vi "Common-AddMsgToListBox.vi"(10 "字符串":string, 11 "列表框":refnum<vi>) -> ()   [LabVIEW 2014]
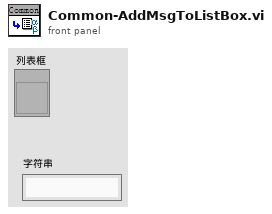
[diagram p1: front panel]
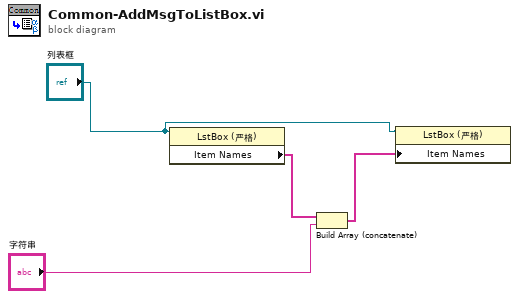
[diagram p0: block diagram]
diagram:
  n1 = property class="LstBox (严格)"(reference="列表框") -> ("Item Names"=w4:string[])  [unwired: 1 in, 2 out]
  n2 = Build Array (concatenate)(w4, "字符串") -> (w2:string[])
  n3 = property class="LstBox (严格)"(reference="列表框", "Item Names"=w2) -> ()  [unwired: 1 in, 2 out]
